vi "GEA2 Write ERD Multiple Messages.vi"(0 "GEA2 Reference In":refnum<k24>, 1 "Retry Count":i32=5, 2 "Read Timeout (ms)":u32=500, 5 "GEA Inputs":T1 {"Destination" format="%.0x"; "Source" format="%.0x"}, 7 "Write ERD List":T2[](array[typedef]) {"ERD Number" format="%.0x"}, 11 "Error In":errorcluster, 12 "#ERDs per message":i32=1 min=1 step=1, 13 "Verify ERD Response?":bool=TRUE) -> (4 "GEA2 Reference Out":refnum<k24>, 8 "Raw Data Out":string[](array[string]), 15 "Error Out":errorcluster)   [LabVIEW 2014, in "GEA2_Toolkit.lvlib"]
uses:
  library/GEA2_Toolkit.lvlib
  type defs/ERD Write Data In.ctl
  C:/Automation/DLLs/PC Tools .NET/GeaCommunication.dll
  Automation/DLLs/PC Tools .NET/GeaCommunication.dll
  type defs/Source_Destination.ctl
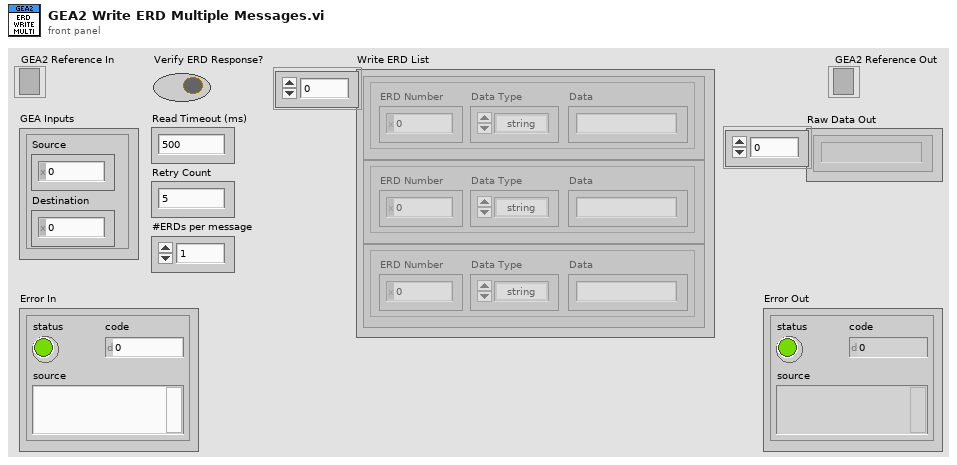
[diagram p1: front panel]
types:
  T1 = typedef "GEA2_Toolkit.lvlib/Source_Destination.ctl" = cluster{"Source":u8, "Destination":u8}
  T2 = typedef "GEA2_Toolkit.lvlib/ERD Write Data In.ctl" = cluster{"ERD Number":u16, "Data Type":enum16{"string", "boolean", "uint8_t", "uint16_t", "uint32_t"}, "Data":string}
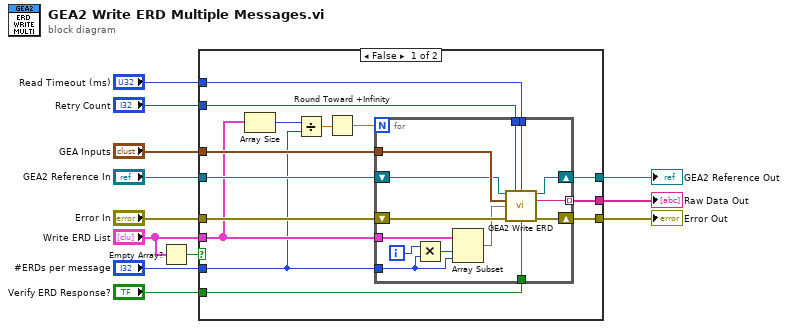
[diagram p0: block diagram]
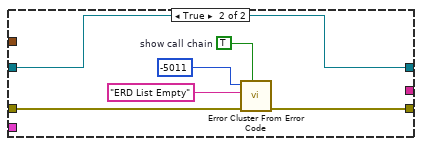
[diagram p2: hidden frame]
diagram:
  n1 = Empty Array?(array="Write ERD List") -> (empty?=w2:bool)
  n2 = case shown="False" w2 {
    tunnel: [w26 w41] -> w12
    tunnel: "Error In" -> [w25 w43]
    tunnel: [w24 w42] -> w10
    tunnel: "Verify ERD Response?" -> [w23 _]
    tunnel: "GEA Inputs" -> [w22 _]
    tunnel: "Read Timeout (ms)" -> [w21 _]
    tunnel: "Retry Count" -> [w20 _]
    tunnel: "GEA2 Reference In" -> [w19 w41]
    tunnel: "Write ERD List" -> [w15 _]
    tunnel: "#ERDs per message" -> [w14 _]
    tunnel: [w13 _] -> w3
    frame False {
      n3 = Array Size(array=w15) -> (size(s)=w18:i32)
      n4 = Divide(x=w18, y=w14) -> (x/y=w17:dbl)
      n5 = Round Toward +Infinity(x=w17) -> (ceil(x): smallest int >= x=w16:dbl)
      n6 = for {
        N: w16 -> [_]
        tunnel: w23 -> [w37]
        tunnel: w22 -> [w36]
        tunnel: [w35] -> w13 mode=indexing
        tunnel: w21 -> [w34]
        tunnel: w20 -> [w33]
        shift-right: [w40] -> w26
        shift-left: w19 -> [w27]
        shift-right: [w38] -> w24
        shift-left: w25 -> [w39]
        tunnel: w15 -> [w32]
        tunnel: w14 -> [w31]
        i -> [w30]
        n7 = Multiply(x=w30, y=w31) -> (x*y=w29:i32)
        n8 = Array Subset(array=w32, index=w29, length=w31) -> (w28:T2[])
        n9 = call "GEA2 Write ERD.vi"("GEA2 Reference In"=w27, "Retry Count"=w33, "Read Timeout (ms)"=w34, "GEA Inputs"=w36, "Write ERD List"=w28, "Error In"=w39, "Verify ERD Response?"=w37) -> ("GEA2 Reference Out"=w40:refnum<k24>, "Raw Data Out"=w35:string, "Error Out"=w38:errorcluster)  [unwired: 6 in]
      }
    }
    frame True {
      w44 = TRUE  # show call chain
      n10 = call <vilib>:"Error Cluster From Error Code.vi"("show call chain? (False)"=w44, "error in (no error)"=w43, "error message (\"\")"="ERD List Empty" ("error message (\"\")"), "error code (0)"=-5011) -> ("error out"=w42:errorcluster)  [unwired: 5 in]
    }
  }
  "GEA2 Reference Out" <- w12
  "Error Out" <- w10
  "Raw Data Out" <- w3
